vi "draw.vi"(0 "reference":refnum<class "SequenceDiagramGraph.lvclass">, 1 "graphics":refnum<class "Graphics.lvclass">, 2 "grid":refnum<class "Grid.lvclass">, 5 "error in (no error)":errorcluster, 6 "SelectedNodes":refnum<class "AbstractNode.lvclass">[](array[class]), 7 "HideOverLays(False)":bool) -> (14 "reference out":refnum<class "SequenceDiagramGraph.lvclass">, 15 "NodesBounds":T4 {"height" format="%.2f"; "width" format="%.2f"; "y" format="%.2f"; "x" format="%.2f"}, 16 "HotSpots":T1[](array[typedef]) {"HotSpot"."y" format="%.2f"; "HotSpot"."x" format="%.2f"}, 19 "error out":errorcluster)   [LabVIEW 2014, in "SequenceDiagramGraph.lvclass"]
doc: "public void draw(Graphics2D g2, Grid g)"
uses:
  <resource>/Framework/Providers/Open_GDS/UML/SequenceDiagramGraph_class/SequenceDiagramGraph.lvclass
  <resource>/Framework/Providers/Open_GDS/UML/Graphics_class/Graphics.lvclass
  <resource>/Framework/Providers/Open_GDS/UML/Grid_class/Grid.lvclass
  <resource>/Framework/Providers/Open_GDS/UML/General/Rectangle/Rectangle Rectangle2D.ctl
  <resource>/Framework/Providers/Open_GDS/UML/AbstractNode_class/AbstractNode.lvclass
  <resource>/Framework/Providers/Open_GDS/UML/UMLEditor/UMLEditor_HotSpotData.ctl
  <resource>/Framework/Providers/Open_GDS/UML/General/Point/Point Point2D.ctl
  <resource>/Framework/Providers/Open_GDS/UML/UMLEditor/UMLEditor_HotSpotType.ctl
  <resource>/Framework/Providers/Open_GDS/UML/AbstractEdge_class/AbstractEdge.lvclass
  <resource>/Framework/Providers/Open_GDS/UML/Graph_class/Graph.lvclass
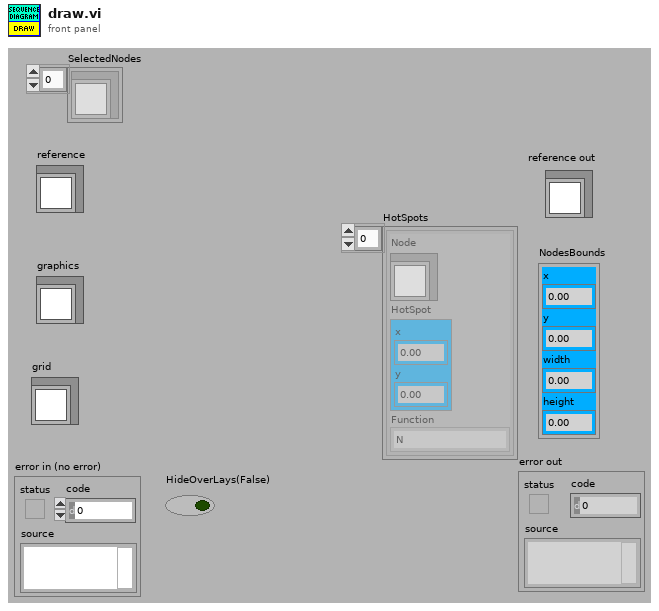
[diagram p1: front panel]
types:
  T1 = typedef "UMLEditor_HotSpotData.ctl" = cluster{"Node":refnum<class "AbstractNode.lvclass">, "HotSpot":T2, "Function":T3}
  T2 = typedef "Point Point2D.ctl" = cluster{"x":dbl, "y":dbl}
  T3 = typedef "UMLEditor_HotSpotType.ctl" = enum16{"N", "NE", "E", "SE", "S", "SW", "W", "NW", "Expand", "Collaps"}
  T4 = typedef "Rectangle Rectangle2D.ctl" = cluster{"x":dbl, "y":dbl, "width":dbl, "height":dbl}
  T5 = typedef "Graph.lvclass/ObjectAttributes.ctl" = cluster{"nodes":refnum<class "AbstractNode.lvclass">[], "edges":refnum<class "AbstractEdge.lvclass">[], "nodesToBeRemoved":refnum<class "AbstractNode.lvclass">[], "edgesToBeRemoved":refnum<class "AbstractEdge.lvclass">[], "needsLayout":bool, "LayoutNodes":refnum<class "AbstractNode.lvclass">[]}
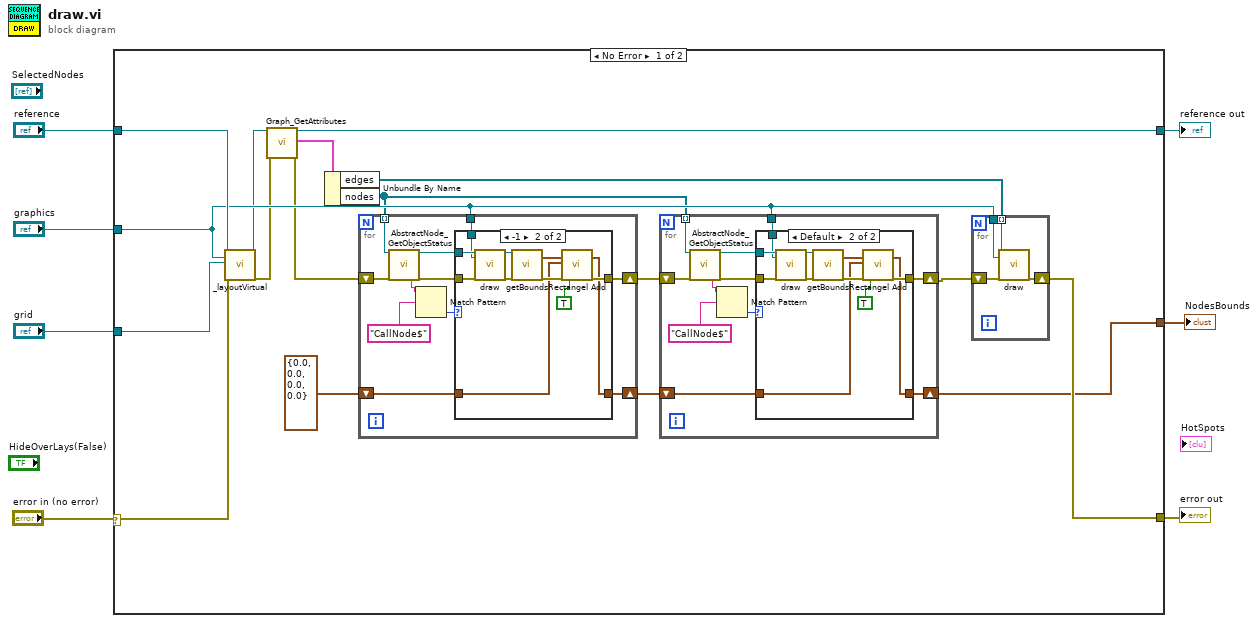
[diagram p0: block diagram]
diagram:
  n1 = case shown="No Error" "error in (no error)" {
    selector: "error in (no error)" -> [w21 w77]
    tunnel: "reference" -> [w24 w78]
    tunnel: [w23 w77] -> w6
    tunnel: [w22 w78] -> w5
    tunnel: "graphics" -> [w20 _]
    tunnel: "grid" -> [w19 _]
    tunnel: [w18 _] -> w1
    frame No Error {
      n2 = call-dynamic "_layoutVirtual.vi"("reference"=w24, "graphics"=w20, "grid"=w19, "error in (no error)"=w21) -> ("reference out"=w16:refnum<class "SequenceDiagramGraph.lvclass">, "error out"=w15:errorcluster)  [unwired: 14 in]
      n3 = call <resource>:"Graph_GetAttributes.vi"("reference in"=w16, "error in (no error)"=w15) -> ("reference out"=w22:refnum<class "SequenceDiagramGraph.lvclass">, "Data"=w8:T5, "error out"=w14:errorcluster)  [unwired: 14 in, 1 out]
      n4 = Unbundle By Name(w8) -> ("edges"=w17:refnum<class "AbstractEdge.lvclass">[], "nodes"=w9:refnum<class "AbstractNode.lvclass">[])
      n5 = for {
        shift-right: [w63] -> w12
        shift-left: w14 -> [w59]
        tunnel: w9 -> [w56] mode=indexing
        tunnel: w20 -> [w54]
        shift-right: [w61] -> w10
        shift-left: T4 {"x"=0.0, "y"=0.0, "width"=0.0, "height"=0.0} ("boundsAdded") -> [w62]
        n6 = call <resource>:"AbstractNode_GetObjectStatus.vi"("reference in"=w56, "error in (no error)"=w59) -> ("Class name"=w53:string, "reference out"=w57:refnum<class "AbstractNode.lvclass">, "error out"=w58:errorcluster)  [unwired: 15 out]
        n7 = Match Pattern(string=w53, regular expression="CallNode$") -> (offset past match=w55:i32)  [unwired: 4 out]
        n8 = case shown="-1" w55 {
          tunnel: [w65 w72] -> w63
          tunnel: w62 -> [w64 w70]
          tunnel: [w64 w69] -> w61
          tunnel: w58 -> [w65 w68]
          tunnel: w57 -> [_ w67]
          tunnel: w54 -> [_ w66]
          frame Default {
          }
          frame -1 {
            n9 = call-dynamic "draw.vi"("reference"=w67, "graphics"=w66, "error in (no error)"=w68) -> ("reference out"=w75:refnum<class "AbstractNode.lvclass">, "error out"=w76:errorcluster)  [unwired: 15 in]
            n10 = call-dynamic "getBounds.vi"("reference"=w75, "error in (no error)"=w76) -> ("bounds"=w74:T4, "error out"=w73:errorcluster)  [unwired: 15 in, 1 out]
            n11 = call <resource>:"Rectangel Add.vi"("bounds1"=w74, "bounds2"=w70, "error in (no error)"=w73, "useAbsoluteCordinates(False)"=TRUE) -> ("boundsAdded"=w69:T4, "error out"=w72:errorcluster)  [unwired: 1 in, 13 out]
          }
        }
      }
      n12 = for {
        shift-right: [w35] -> w11
        shift-left: w12 -> [w31]
        tunnel: w9 -> [w28] mode=indexing
        tunnel: w20 -> [w26]
        shift-right: [w33] -> w18
        shift-left: w10 -> [w34]
        n13 = call <resource>:"AbstractNode_GetObjectStatus.vi"("reference in"=w28, "error in (no error)"=w31) -> ("Class name"=w25:string, "reference out"=w29:refnum<class "AbstractNode.lvclass">, "error out"=w30:errorcluster)  [unwired: 15 out]
        n14 = Match Pattern(string=w25, regular expression="CallNode$") -> (offset past match=w27:i32)  [unwired: 4 out]
        n15 = case shown="Default" w27 {
          tunnel: [w37 w44] -> w35
          tunnel: w34 -> [w36 w42]
          tunnel: [w36 w41] -> w33
          tunnel: w30 -> [w37 w40]
          tunnel: w29 -> [_ w39]
          tunnel: w26 -> [_ w38]
          frame -1 {
          }
          frame Default {
            n16 = call-dynamic "draw.vi"("reference"=w39, "graphics"=w38, "error in (no error)"=w40) -> ("reference out"=w47:refnum<class "AbstractNode.lvclass">, "error out"=w48:errorcluster)  [unwired: 15 in]
            n17 = call-dynamic "getBounds.vi"("reference"=w47, "error in (no error)"=w48) -> ("bounds"=w46:T4, "error out"=w45:errorcluster)  [unwired: 15 in, 1 out]
            n18 = call <resource>:"Rectangel Add.vi"("bounds1"=w46, "bounds2"=w42, "error in (no error)"=w45, "useAbsoluteCordinates(False)"=TRUE) -> ("boundsAdded"=w41:T4, "error out"=w44:errorcluster)  [unwired: 1 in, 13 out]
          }
        }
      }
      n19 = for {
        shift-right: [w51] -> w23
        shift-left: w11 -> [w52]
        tunnel: w17 -> [w49] mode=indexing
        tunnel: w20 -> [w50]
        n20 = call-dynamic "draw.vi"("reference"=w49, "graphics"=w50, "error in (no error)"=w52) -> ("error out"=w51:errorcluster)  [unwired: 15 in, 1 out]
      }
    }
    frame Error {
    }
  }
  "reference out" <- w5
  "error out" <- w6
  "NodesBounds" <- w1
